vi "Window_Expend.vi"(8 "error in (no error)":errorcluster, 10 "height":i16, 11 "width":i16) -> (0 "error out":errorcluster)   [LabVIEW 2019]
uses:
  <vilib>/Utility/miscctls.llb/LVRectTypeDef.ctl
panel:
  # "input"
  # "ouput"
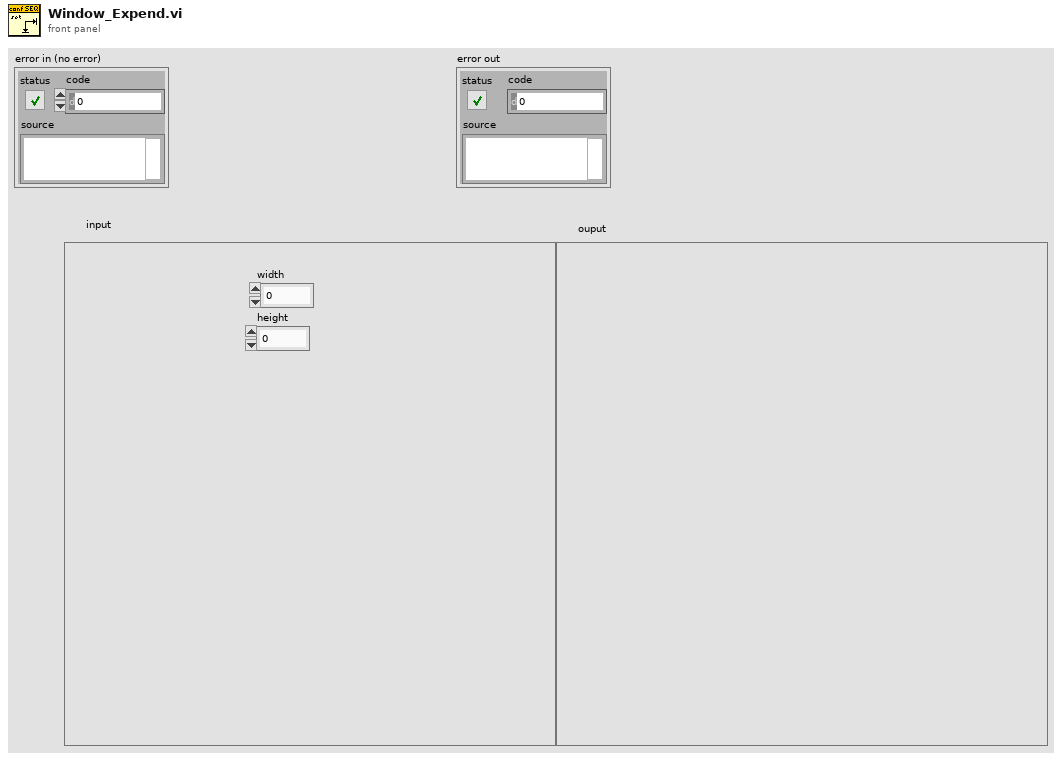
[diagram p1: front panel]
types:
  T1 = typedef "LVRectTypeDef.ctl" = cluster{"Left":i16, "Top":i16, "Right":i16, "Bottom":i16}
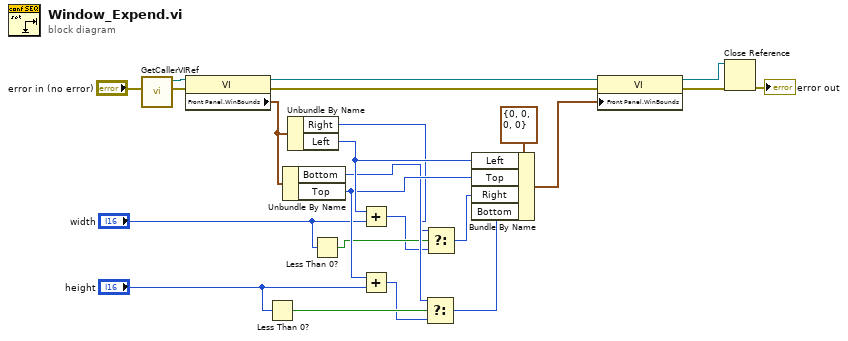
[diagram p0: block diagram]
diagram:
  n1 = call "GetCallerVIRef.vi"("error in (no error)"="error in (no error)") -> ("error out"=w12:errorcluster, "VI out"=w11:refnum<vi>)  [unwired: 9 in]
  n2 = property class="VI"(reference=w11, error in=w12) -> (reference out=w22:refnum<vi>, error out=w15:errorcluster, "Front Panel.WinBounds"=w23:T1)
  n3 = Less Than 0?(x="height") -> (x < 0?=w9:bool)
  n4 = Unbundle By Name(w23) -> ("Bottom"=w6:i16, "Top"=w18:i16)
  n5 = Unbundle By Name(w23) -> ("Right"=w1:i16, "Left"=w19:i16)
  n6 = Less Than 0?(x="width") -> (x < 0?=w4:bool)
  n7 = Add(x=w19, y="width") -> (x+y=w3:i16)
  n8 = Add(x=w18, y="height") -> (x+y=w8:i16)
  n9 = Select(t=w6, s=w9, f=w8) -> (s? t:f=w7:i16)
  n10 = Select(t=w1, s=w4, f=w3) -> (s? t:f=w2:i16)
  n11 = Bundle By Name(cluster=T1 {"Left"=0, "Top"=0, "Right"=0, "Bottom"=0} ("Front Panel Window:Window Bounds"), "Left"=w19, "Top"=w18, "Right"=w2, "Bottom"=w7) -> (w20:T1)
  n12 = property class="VI"(reference=w22, error in=w15, "Front Panel.WinBounds"=w20) -> (reference out=w16:refnum<vi>, error out=w17:errorcluster)
  n13 = Close Reference(reference=w16, error in (no error)=w17) -> (error out=→"error out":errorcluster)
